vi "Delete IPF.vi"(8 "error in":errorcluster, 9 "APG Config":T1, 10 "Programs List":i32(listbox)) -> (0 "error out":errorcluster, 2 "Programs List":i32(listbox))   [LabVIEW 2013, in "Manipulate IPF.lvlib"]
uses:
  Manipulate IPF.lvlib
  Settings/type_def/APG Config.ctl
  <userlib>/_OpenG.lib/file/file.llb/Strip Path Extension - String__ogtk.vi
  <userlib>/_OpenG.lib/file/file.llb/Convert File Extension (String)__ogtk.vi
  Settings/APG_settings.lvlib
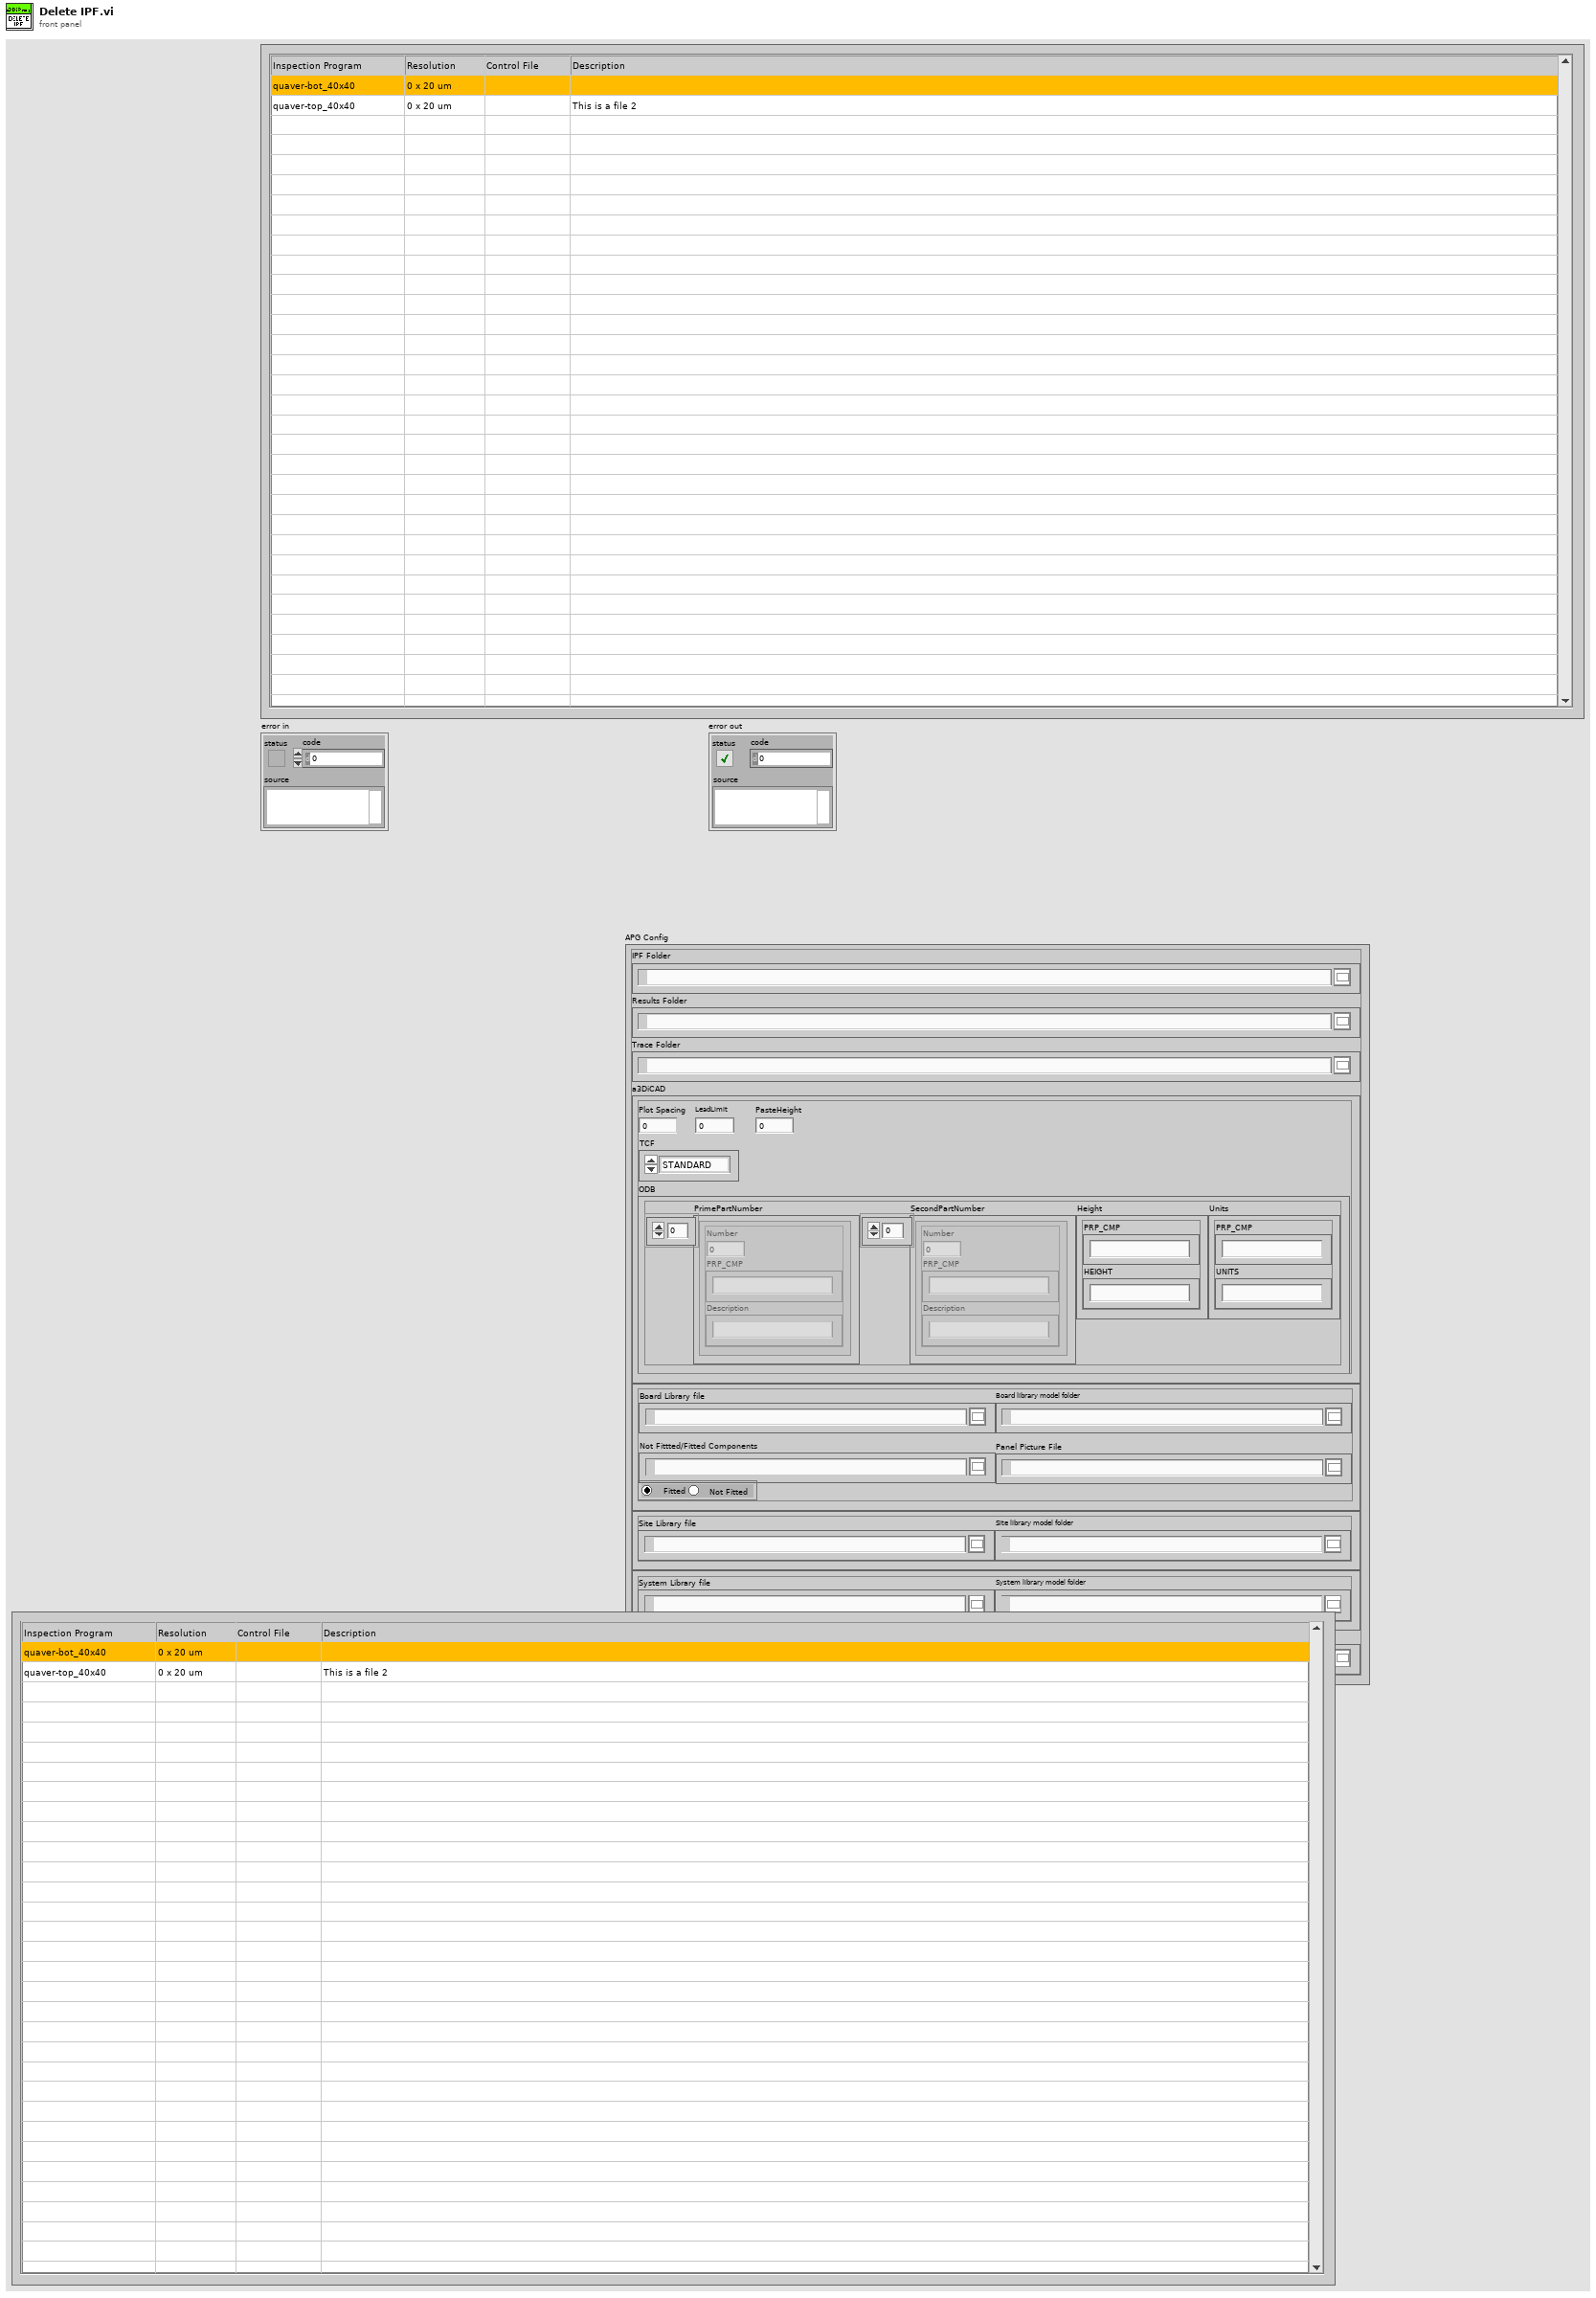
[diagram p1: front panel]
types:
  T1 = typedef "APG_settings.lvlib/APG Config.ctl" = cluster{"IPF Folder":path, "Results Folder":path, "Trace Folder":path, "a3DiCAD":cluster{"Plot Spacing":dbl, "TCF":enum16{"STANDARD", "PASTE", "LEAD"}, "LeadLimit":u32, "a3DiCADDebug":bool, "ODB":cluster{"PrimePartNumber":cluster{"Number":u32, "PRP_CMP":string, "Description":string}[], "SecondPartNumber":cluster{"Number":u32, "PRP_CMP":string, "Description":string}[], "Height":cluster{"PRP_CMP":string, "HEIGHT":string}, "Units":cluster{"PRP_CMP":string, "UNITS":string}}, "PasteHeight":dbl}, "a3DiCADcfg":path, "Board Library":cluster{"Board Library file":path, "Board library model folder":path, "Not Fittted/Fitted Components":path, "Panel Picture File":path, "Components":enum32{"Fitted", "Not Fitted "}}, "Site Library":cluster{"Site Library file":path, "Site library model folder":path}, "System Library":cluster{"System Library file":path, "System library model folder":path}, "ODB++ file":path}
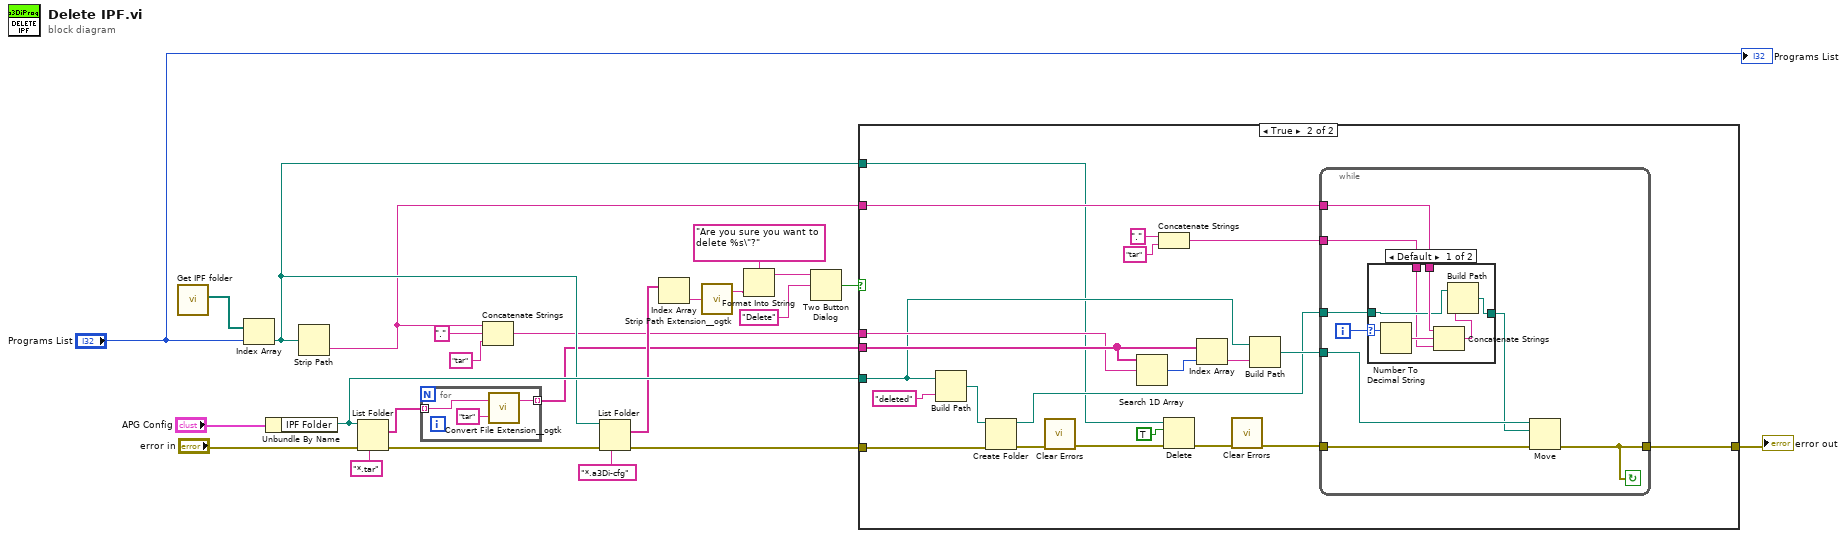
[diagram p0: block diagram]
diagram:
  n1 = call "Get IPF folder.vi"() -> ("IPF sub folders"=w22:path[])  [unwired: 6 in, 5 out]
  n2 = Index Array(array=w22, index="Programs List") -> (element=w12:path)
  n3 = Unbundle By Name("APG Config") -> ("IPF Folder"=w17:path)
  n4 = Strip Path(path=w12) -> (name=w2:string)  [unwired: 1 out]
  n5 = List Folder(path=w17, pattern="*.tar", error in="error in") -> (filenames=w6:string[], error out=w14:errorcluster)  [unwired: 1 in, 2 out]
  n6 = for {
    tunnel: [w27] -> w5 mode=indexing
    tunnel: w6 -> [w26] mode=indexing
    n7 = call-poly <userlib>:"Convert File Extension__ogtk.vi"("new ending (none)"="tar", "file name"=w26) -> ("new filename"=w27:string)  [unwired: 1 out]
  }
  n8 = Concatenate Strings(w2, "." ("string"), "tar" ("new ending (none)")) -> (w1:string)
  n9 = List Folder(path=w12, pattern="*.a3Di-cfg", error in=w14) -> (filenames=w9:string[], error out=w13:errorcluster)  [unwired: 1 in, 2 out]
  n10 = Index Array(array=w9) -> (element=w8:string)  [unwired: 1 in]
  n11 = call-poly <userlib>:"Strip Path Extension__ogtk.vi"("path"=w8) -> ("root"=w7:string)  [unwired: 1 out]
  n12 = Format Into String(format string="Are you sure you want to delete %s\"?", w7) -> (resulting string=w20:string)  [unwired: 2 in, 1 out]
  n13 = Two Button Dialog(message=w20, 2:"Delete" ("T button name (\"OK\")")) -> (T button?=w18:bool)  [unwired: 1 in]
  n14 = case shown="True" w18 {
    tunnel: w13 -> [w28 w44]
    tunnel: w17 -> [_ w41]
    tunnel: w5 -> [_ w43]
    tunnel: w1 -> [_ w42]
    tunnel: [w28 w34] -> w16
    tunnel: w2 -> [_ w38]
    tunnel: w12 -> [_ w29]
    frame False {
    }
    frame True {
      n15 = Build Path(base path=w41, name or relative path="deleted") -> (appended path=w47:path)
      n16 = Create Folder(path (use dialog)=w47, error in=w44) -> (created path=w39:path, error out=w46:errorcluster)  [unwired: 1 in, 1 out]
      n17 = call <vilib>:"Clear Errors.vi"("error in (no error)"=w46) -> ("error out"=w33:errorcluster)  [unwired: 6 in]
      n18 = Search 1D Array(1D array=w43, element=w42) -> (index of element=w48:i32)  [unwired: 1 in]
      n19 = Concatenate Strings("." ("string"), "tar" ("new ending (none)")) -> (w36:string)
      n20 = Delete(path (use dialog)=w29, entire hierarchy (F)=TRUE, error in=w33) -> (error out=w32:errorcluster)  [unwired: 2 in, 2 out]
      n21 = Index Array(array=w43, index=w48) -> (element=w49:string)
      n22 = call <vilib>:"Clear Errors.vi"("error in (no error)"=w32) -> ("error out"=w31:errorcluster)  [unwired: 6 in]
      n23 = Build Path(base path=w41, name or relative path=w49) -> (appended path=w40:path)
      n24 = while {
        tunnel: w40 -> [w57]
        tunnel: w31 -> [w56]
        tunnel: [w50] -> w34
        tunnel: w39 -> [w53]
        tunnel: w38 -> [w52]
        tunnel: w36 -> [w51]
        i -> [w55]
        stop <- w50 continue-if-true
        n25 = case shown="Default" w55 {
          selector: w55 -> [w64 _]
          tunnel: [w61 w65] -> w54
          tunnel: w52 -> [w62 _]
          tunnel: w53 -> [w59 w65]
          tunnel: w51 -> [w58 _]
          frame Default {
            n26 = Number To Decimal String(number=w64) -> (decimal integer string=w63:string)  [unwired: 1 in]
            n27 = Concatenate Strings(w62, w63, w58) -> (w60:string)
            n28 = Build Path(base path=w59, name or relative path=w60) -> (appended path=w61:path)
          }
          frame 0 {
          }
        }
        n29 = Move(source path=w57, error in=w56, 10:w54) -> (error out=w50:errorcluster)  [unwired: 2 in, 2 out]
      }
    }
  }
  "error out" <- w16
  "Programs List" <- "Programs List"
